vi "sm i16 read array and increment.vi"(8 "error in (no error)":errorcluster, 9 "array size":i64, 10 "increment value":u64=2, 11 "pointer in":u64) -> (0 "error out":errorcluster, 2 "value out":i16[](array[numeric]), 3 "Shared Memory PTR out":u64)   [LabVIEW 2018, in "linuxSharedMemory.lvlib"]
uses:
  linuxSharedMemory.lvlib
  <vilib>/NI/NI Linux RT IPC/Shared Memory/Pointer Operations/Read 1D Array I16.vi
  <vilib>/NI/NI Linux RT IPC/Shared Memory/Pointer Operations/In Place Read 1D Array I16.vi
  <vilib>/NI/NI Linux RT IPC/Shared Memory/Linux RT IPC.Shared Memory.lvlib
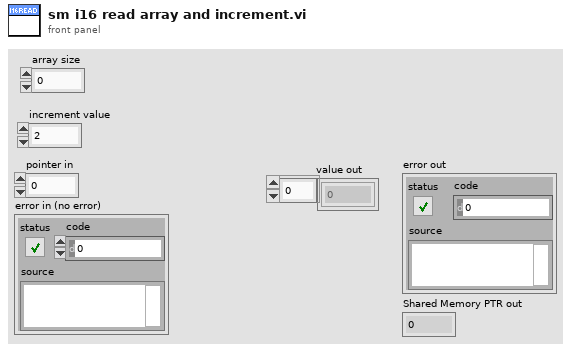
[diagram p1: front panel]
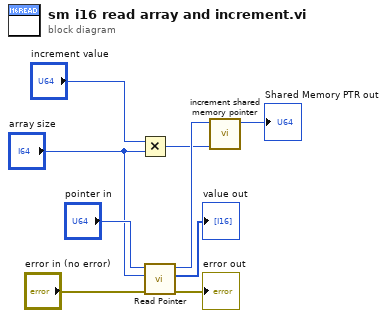
[diagram p0: block diagram]
diagram:
  n1 = Multiply(x="increment value", y="array size") -> (x*y=w1:u64)
  n2 = call-poly <vilib>:"Read Pointer.vi"("error in (no error)"="error in (no error)", "number of elements"="array size", "pointer in"="pointer in") -> ("error out"=→"error out":errorcluster, "value"=→"value out":i16[], "pointer out"=w9:u64)  [unwired: 5 in, 1 out]
  n3 = call "increment shared memory pointer.vi"("Increment value"=w1, "Shared Memory PTR in"=w9) -> ("Shared Memory PTR out"=→"Shared Memory PTR out":u64)  [unwired: 9 in]
